vi "Check Special Condition.vi"(7 "Current Cond":T1, 8 "Error In":errorcluster, 9 "Full Cutout?":bool, 10 "Trigger Draw":bool, 11 "Station Data Input":T2={"Sequence #"=0.0, "Cycles"=0, "Mode Setting"="", "Flow Rate (GPM)"=0.0, "Temperature (F)"=0.0, "Reset Timer"=FALSE, "Use Temp Decline Method"=FALSE, "Terminate Condition"=enum."C1-Terminate Draw @ Gallon Mark", "Condition Value #1"=0.0, "UE"=FALSE, "LE"=FALSE, "Comp"=FALSE, "Fan"=FALSE, "Test End Time (Sec)"=0.0, "Purge Until Cutout"=FALSE, "Start Conditions"=enum."Heat Source Cutout", "Condition Value #2"=0.0, "Remove Power"=FALSE, "Time"=0.0, "Check Special Cond."=enum."SC2-Check Heat Source (On-C2/Off-C1)", "Condition#"=enum."C1", "Draw Flags"=enum."N/A", "Data Processing Delay (FHD 15sec, UEF 5 Sec)"=0.0, "Test Complete"=FALSE} {"Time" format="%<%H:%M:%S>t"}) -> (0 "Error Out":errorcluster, 2 "Trigger Draw Out":bool, 3 "Condition":T1)   [LabVIEW 2016]
uses:
  Type Definitions/HEWH Special Condition Check.ctl
  Type Definitions/PRAT Test.ctl
  Utility/Save File/File Setup (Public)/Type Definition/Save File HEWH Heating Control Mode.ctl
  Type Definitions/Terminate Draw Conditions.ctl
  Type Definitions/HEWH Start Conditions.ctl
  Type Definitions/Check Special Condtions.ctl
  Type Definitions/HEWH Draw Flag ENUM.ctl
  Utility/Save File/File Setup.lvlib
panel:
  out "Saved Condition Read":T1
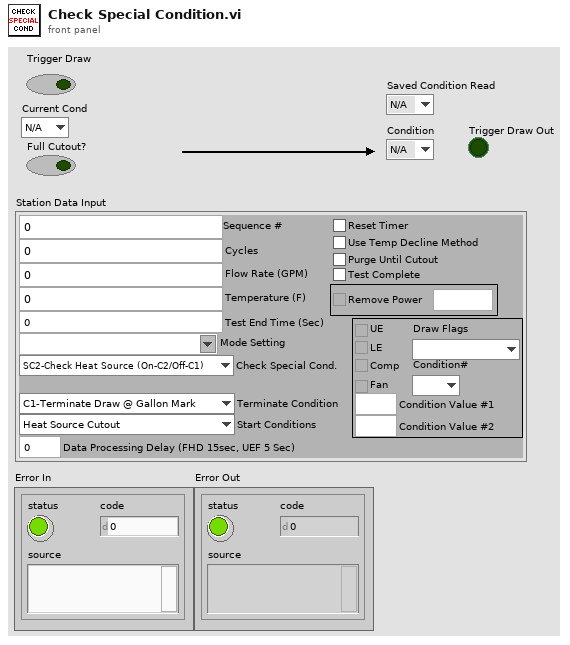
[diagram p1: front panel]
types:
  T1 = typedef "HEWH Special Condition Check.ctl" = enum16{"N/A", "C1", "C2", "Reset/Fail", "Skip Draw Sequence"}
  T2 = typedef "PRAT Test.ctl" = cluster{"Sequence #":dbl, "Cycles":i32, "Mode Setting":T3, "Flow Rate (GPM)":dbl, "Temperature (F)":dbl, "Reset Timer":bool, "Use Temp Decline Method":bool, "Terminate Condition":T4, "Condition Value #1":dbl, "UE":bool, "LE":bool, "Comp":bool, "Fan":bool, "Test End Time (Sec)":dbl, "Purge Until Cutout":bool, "Start Conditions":T5, "Condition Value #2":dbl, "Remove Power":bool, "Time":dbl, "Check Special Cond.":T6, "Condition#":T1, "Draw Flags":T7, "Data Processing Delay (FHD 15sec, UEF 5 Sec)":dbl, "Test Complete":bool}
  T3 = typedef "File Setup.lvlib/Save File HEWH Heating Control Mode.ctl" = string
  T4 = typedef "Terminate Draw Conditions.ctl" = enum16{"C1-Terminate Draw @ Gallon Mark", "C2-Special Last Draw (HU Test)", "C3-RTD Out <=", "C4-Mean Tank Temp <=", "C5-Decrease RTD Out (Deg F)", "C6-Time (Seconds)", "C7-Until Any Heat Source", "C8-Specific Heat Source", "C9-Do Nothing"}
  T5 = typedef "HEWH Start Conditions.ctl" = enum16{"Heat Source Cutout", "At Time (Seconds)", "Every X (Seconds)", "T2 >= X° Below Setpoint", "Seconds From Complete", "Wait for LE & Comp Cutout", "Wait for Comp Cutout", "Wait for LE Cutout", "Wait for UE Cutout"}
  T6 = typedef "Check Special Condtions.ctl" = enum16{"SC1-Do Nothing", "SC2-Check Heat Source (On-C2/Off-C1)", "SC3-Check Skip Condition", "SC4-Check Heat Source ON/Fail"}
  T7 = typedef "HEWH Draw Flag ENUM.ctl" = enum16{"N/A", "None(0)", "Sml(1)", "Med(2)", "SmlMed(3)", "Lrg(4)", "SmlLrg(5)", "MedLrg(6)", "SmlMedLrg(7)"}
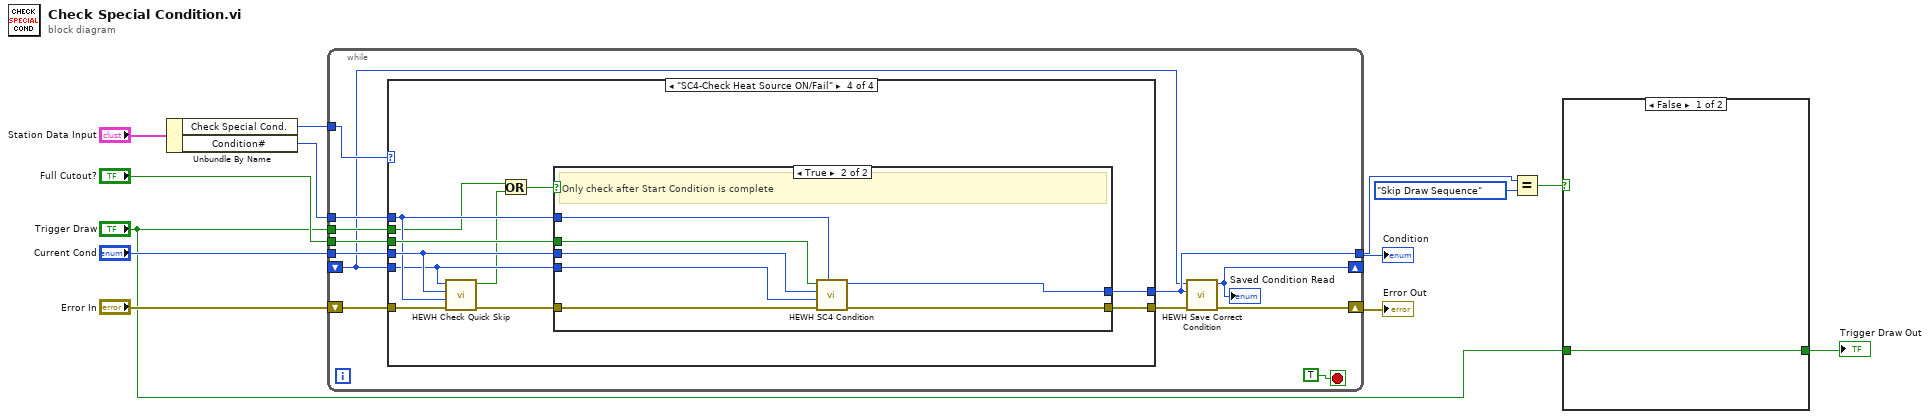
[diagram p0: block diagram]
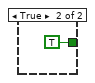
[diagram p2: hidden frame]
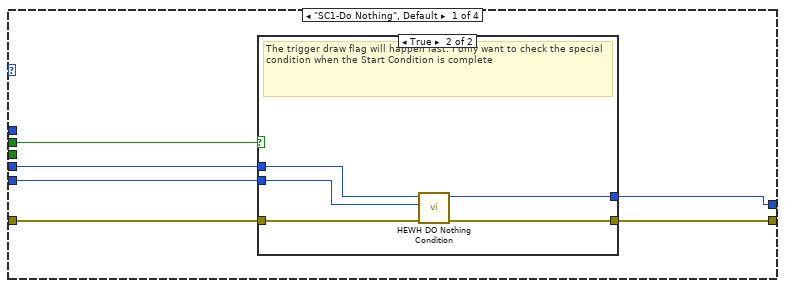
[diagram p3: hidden frame]
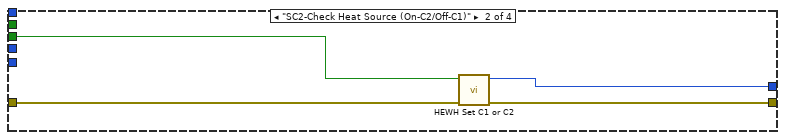
[diagram p5: hidden frame]
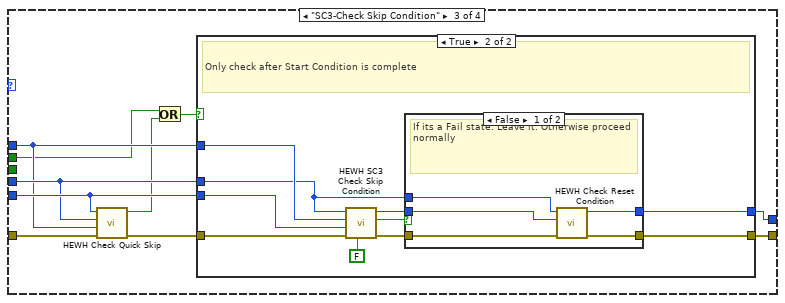
[diagram p6: hidden frame]
diagram:
  n1 = Unbundle By Name("Station Data Input") -> ("Check Special Cond."=w10:T6, "Condition#"=w6:T1)
  n2 = while {
    tunnel: "Full Cutout?" -> [w24]
    tunnel: w10 -> [w23]
    tunnel: "Current Cond" -> [w22]
    tunnel: [w17] -> w5
    tunnel: w6 -> [w21]
    tunnel: "Trigger Draw" -> [w19]
    shift-right: [w14] -> w7
    shift-left: "Error In" -> [w20]
    shift-right: [w16] -> _
    shift-left: _ -> [w13]
    stop <- TRUE stop-if-true
    n3 = case shown="\"SC4-Check Heat Source ON/Fail\"" w23 {
      tunnel: w24 -> [_ w41 _ w80]
      tunnel: [w27 w40 w51 w81] -> w17
      tunnel: w22 -> [w26 _ w46 w78]
      tunnel: w21 -> [_ _ w45 w77]
      tunnel: w20 -> [w30 w39 w49 w75]
      tunnel: [w29 w38 w50 w79] -> w15
      tunnel: w19 -> [w25 _ w44 w73]
      tunnel: w13 -> [w28 _ w47 w76]
      frame "SC1-Do Nothing", Default {
        n4 = case shown="True" w25 {
          tunnel: w30 -> [w32 w37]
          tunnel: [w32 w36] -> w29
          tunnel: w28 -> [_ w35]
          tunnel: [w31 w34] -> w27
          tunnel: w26 -> [w31 w33]
          frame False {
          }
          frame True {
            # "The trigger draw flag will happen last. I only want to check the special condition when the Start Condition is complete"
            n5 = call "HEWH DO Nothing Condition.vi"("error in (no error)"=w37, "Saved Condition"=w35, "Current Cond"=w33) -> ("error out"=w36:errorcluster, "Current Cond Out"=w34:T1)  [unwired: 7 in]
          }
        }
      }
      frame "SC2-Check Heat Source (On-C2/Off-C1)" {
        n6 = call "HEWH Set C1 or C2.vi"("Error In"=w39, "Full Cutout?"=w41) -> ("Error Out"=w38:errorcluster, "Current Cond Out"=w40:T1)  [unwired: 8 in]
      }
      frame "SC3-Check Skip Condition" {
        n7 = call "HEWH Check Quick Skip.vi"("Error In"=w49, "Condition#"=w45, "Current Cond"=w46, "Saved Condition Read"=w47) -> ("Error Out"=w48:errorcluster, "Quick Skip?"=w43:bool)  [unwired: 6 in]
        n8 = Or(x=w44, y=w43) -> (x .or. y?=w42:bool)
        n9 = case shown="True" w42 {
          tunnel: w45 -> [_ w63]
          tunnel: [w52 w56] -> w51
          tunnel: w47 -> [_ w55]
          tunnel: w48 -> [w53 w62]
          tunnel: [w53 w60] -> w50
          tunnel: w46 -> [w52 w57]
          frame False {
          }
          frame True {
            # "Only check after Start Condition is complete"
            n10 = call "HEWH SC3 Check Skip Condition.vi"("Use Current Cond?"=FALSE, "Error In"=w62, "Saved Condition"=w55, "Condition#"=w63, "Current Cond"=w57) -> ("Error Out"=w61:errorcluster, "Conditions Equal?"=w59:bool, "SC3 Check Skip"=w58:T1)  [unwired: 4 in]
            n11 = case shown="False" w59 {
              tunnel: w61 -> [w68 w69]
              tunnel: [w67 w69] -> w60
              tunnel: w58 -> [w66 w70]
              tunnel: w57 -> [w65 _]
              tunnel: [w64 w70] -> w56
              frame False {
                # "If its a Fail state. Leave it. Otherwise proceed normally"
                n12 = call "HEWH Check Reset Condition.vi"("Error In"=w68, "SC3 Check Skip"=w66, "Current Cond"=w65) -> ("Error Out"=w67:errorcluster, "Current Cond"=w64:T1)  [unwired: 6 in, 1 out]
              }
              frame True {
              }
            }
          }
        }
      }
      frame "SC4-Check Heat Source ON/Fail" {
        n13 = call "HEWH Check Quick Skip.vi"("Error In"=w75, "Condition#"=w77, "Current Cond"=w78, "Saved Condition Read"=w76) -> ("Error Out"=w74:errorcluster, "Quick Skip?"=w72:bool)  [unwired: 6 in]
        n14 = Or(x=w73, y=w72) -> (x .or. y?=w71:bool)
        n15 = case shown="True" w71 {
          tunnel: [w83 w90] -> w81
          tunnel: w80 -> [_ w89]
          tunnel: w78 -> [w83 w88]
          tunnel: w74 -> [w82 w87]
          tunnel: [w82 w86] -> w79
          tunnel: w77 -> [_ w85]
          tunnel: w76 -> [_ w84]
          frame False {
          }
          frame True {
            # "Only check after Start Condition is complete"
            n16 = call "HEWH SC4 Condition.vi"("Condition#"=w85, "Error In"=w87, "Saved Condition"=w84, "Current Cond"=w88, "Full Cutout?"=w89) -> ("Error Out"=w86:errorcluster, "Current Cond Out"=w90:T1)  [unwired: 5 in]
          }
        }
      }
    }
    n17 = call "HEWH Save Correct Condition.vi"("Error In"=w15, "Current Cond"=w17, "Saved Condition"=w13) -> ("Error Out"=w14:errorcluster, "Saved Condition Read"=w16:T1)  [unwired: 7 in]
    "Saved Condition Read" <- w16
  }
  "Error Out" <- w7
  "Condition" <- w5
  n18 = Equal?(x=w5, y=HEWH_Special_Condition_Check."Skip Draw Sequence") -> (x = y?=w3:bool)
  n19 = case shown="False" w3 {
    tunnel: "Trigger Draw" -> [w91 _]
    tunnel: [w91 TRUE ("Trigger Draw")] -> w1
    frame False {
    }
    frame True {
    }
  }
  "Trigger Draw Out" <- w1
